vi "MFLI controller -- via frontend -- V2.vi"(1 "MFLI controller action":T1=enum."Scan frequency", 5 "Address":string="DEV3523", 9 "sweep parameters":T2={"scan type"=enum."arctan", "N"=100, "cursor window"={"left"=32571.699125630872, "right "=32589.533031344432, "center"=32580.616078487652, "window"=17.83390571355876, "cursors"=[0, 1, 2], "relative"=0, "absolute"=0, "fixed vertical offset"=0.0, "vertical offset"=0.0, "skew"=0.0, "default window frac"=0.1, "kind"=enum."symmetric", "skew.left"=0.5, "skew.right"=0.5, "Plot ref"=refnum, "wing order"=enum."forw"}}, 11 "Error In":errorcluster, 12 "reqested size":i32=100, 13 "delay (msec)":i64=2) -> (4 "Freq out (Hz)":dbl[](array[numeric])=[32012.991918577427, 32390.261658505893, 32466.39798177853, 32499.14340521798, 32517.39286113775, 32529.046092051318, 32537.14525712326, 32543.111142615544, 32547.696343954158, 32551.33675949651, 32554.302325209504, 32556.769142360055, 32558.856995237307, 32560.650202739795, 32562.209843476354, 32563.58125099723, 32564.7987833122, 32565.88895894197, 32566.872575330308, 32567.766175404246, 32568.583086316496, 32569.334166794306, 32570.02835688638, 32570.673085530187, 32571.274580490695, 32571.838104118455, 32572.36813539066, 32572.868514009202, 32573.342552524307, 32573.793126289274, 32574.222746575288, 32574.633618125405, 32575.027687968828, 32575.40668442971, 32575.772149741057, 32576.12546690325, 32576.467883345118, 32576.800529469096, 32577.124435064776, 32577.440543590797, 32577.749724325146, 32578.052781957467, 32578.35046682089, 32578.643482565894, 32578.932492128843, 32579.218126471686, 32579.500987779396, 32579.781656707495, 32580.06069600583, 32580.338656060805, 32580.616078519142, 32580.89350097748, 32581.171461032456, 32581.45050033079, 32581.73116925889, 32582.0140305666, 32582.29966469628, 32582.58867447239, 32582.88169000423, 32583.179375080817, 32583.48243271314, 32583.791613234323, 32584.10772197351, 32584.43162756919, 32584.764273480003, 32585.106690135035, 32585.460007297228, 32585.825472395412, 32586.204468856296, 32586.59853891288, 32587.009410462997, 32587.439030535847, 32587.889604513977, 32588.363642815923, 32588.86402143446, 32589.39405291983, 32589.957576334426, 32590.559071508098, 32591.203800151903, 32591.897990030815, 32592.64907072179, 32593.46598163404, 32594.359581707977, 32595.343197883154, 32596.433373726086, 32597.650906041054, 32599.022313348767, 32600.58195429849, 32602.375161800977, 32604.46301467823, 32606.929831615616, 32609.895397541775, 32613.535812870963, 32618.12101442274, 32624.086899701866, 32632.186064986967, 32643.839295900536, 32662.088751820305, 32694.834175046595, 32770.97049853239], 6 "sweep time":dbl=1.133070214302279, 10 "Voltage out (V)":cdb[](array[numeric])=[1.7183506006211996e-05-0.0001154032788780638i, 1.7124360968751133e-05-0.0001154114779288915i, 1.7049104347380084e-05-0.00011541542942613611i, 1.700437896335042e-05-0.00011541749156201827i, 1.6984579723285106e-05-0.00011542204741013496i, 1.702277369054923e-05-0.00011543195548892015i, 1.713094025845651e-05-0.00011543928112855599i, 1.734249707866828e-05-0.00011543960094139092i, 1.768320429215342e-05-0.0001154245402225022i, 1.8195281152538477e-05-0.00011538335923575508i, 1.8917228661806973e-05-0.00011530288392402138i, 1.9897834564883332e-05-0.00011516640933089982i, 2.154104046962704e-05-0.0001148906117047364i, 2.3247799321765792e-05-0.00011455940834964969i, 2.5364678450551808e-05-0.00011410149936074356i, 2.8645788781885885e-05-0.00011331572480450341i, 3.204749554800641e-05-0.00011242961468546203i, 3.783559691555022e-05-0.00011080033368711338i, 4.245015867332296e-05-0.00010941815048749576i, 4.909131821431355e-05-0.0001073312840925185i, 5.511821898441184e-05-0.00010535829212367013i, 6.178843506022867e-05-0.00010310289174359778i, 7.1079604965352e-05-9.985157907779013e-05i, 7.922304381453334e-05-9.690255343156676e-05i, 8.814778883893872e-05-9.35627973091444e-05i, 9.806709148886077e-05-8.971246458508318e-05i, 0.00011119043245647465-8.437841897470898e-05i, 0.00012253184919712196-7.953180105990741e-05i, 0.00013777724317049346-7.26422052575784e-05i, 0.0001508081004573332-6.638511645494567e-05i, 0.00016547294918783876-5.890291826790314e-05i, 0.00018003847596605868-5.097295421607585e-05i, 0.00019518361086534857-4.2160672625888326e-05i, 0.00021134179818259658-3.207632261667366e-05i, 0.0002372041782935464-1.434566976209705e-05i, 0.00025518143132024254-7.65423157605567e-07i, 0.0002835129702467886+2.297908707067173e-05i, 0.0003060118087631287+4.414715126576145e-05i, 0.00032860772064336976+6.780161699354136e-05i, 0.0003492674091322389+9.188627597766353e-05i, 0.00037498324855458583+0.0001258445655672888i, 0.00040021078021115026+0.00016463936720210011i, 0.00041969942568205823+0.0001996255883353531i, 0.00044367338947118773+0.00025154867300893595i, 0.0004634793607238068+0.0003068834938295352i, 0.00047921028781215815+0.00036805191402776324i, 0.0004880906353641744+0.00042166295770603194i, 0.0004932212623741357+0.0004947057496862386i, 0.000491476456593048+0.0005562791342814882i, 0.000480893803992059+0.0006363872629062725i, 0.0004535995818650303+0.0007373086546111893i, 0.000417087772881063+0.0008226852134031236i, 0.0003564148692854789+0.0009214817173403453i, 0.0003049201646356487+0.0009841224100520793i, 0.00021260191240459413+0.0010684135492785532i, 0.00011714858948470126+0.001130293664798013i, 1.675457544365132e-05+0.0011752384955043165i, -6.8674075405897e-05+0.0012001399159748158i, -0.000156473047607305+0.0012143601357779102i, -0.00026709373934749337+0.0012167952520739987i, -0.0003544271565676041+0.001206585218500233i, -0.00047937600197311275+0.0011721904461218277i, -0.0006086290582260493+0.0011080263068835828i, -0.0007031877411848573+0.0010369948237613604i, -0.0007564526901441745+0.0009845652865779295i, -0.000802489180995596+0.0009292050493656664i, -0.0008414596018105983+0.0008721985101652608i, -0.0008809346482248761+0.0008000538120167723i, -0.0009073902840241921+0.0007382113118499092i, -0.0009264953054508651+0.000680980624166274i, -0.0009405659412141811+0.0006247883223244968i, -0.000951649722530156+0.0005564170049287236i, -0.0009557485581057351+0.0005027508202624884i, -0.0009558464741053665+0.0004515634249715623i, -0.0009509110176922098+0.0003899637122391104i, -0.0009411315169847015+0.00033238768338539245i, -0.0009303400913929496+0.0002890952314710416i, -0.0009171113529290538+0.00024772942260094455i, -0.0009022111527275027+0.00020961974320628598i, -0.0008813746494947608+0.00016554205395646727i, -0.0008581837971946129+0.00012481593212717478i, -0.0008372063466683705+9.328565348151487e-05i, -0.0008165626610594428+6.595676342721183e-05i, -0.0007901155435838691+3.51376371228606e-05i, -0.0007682834352800848+1.2585785624721776e-05i, -0.000746231015527196-7.956667433689733e-06i, -0.0007238798463130141-2.6771164006128246e-05i, -0.0007015567569177018-4.3779400880525094e-05i, -0.000679301954671598-5.9154880569231366e-05i, -0.0006572001413831251-7.301304884663801e-05i, -0.000629855254567978-8.838260380910578e-05i, -0.0006083942229188815-9.917719243438264e-05i, -0.0005768631156754208-0.00011317657292622015i, -0.0005562177438951648-0.00012121832857134644i, -0.0005359092039599222-0.00012831021292074535i, -0.0005145186443378148-0.00013494179211461784i, -0.0004951602053444319-0.00014023403510992087i, -0.00047624970229075174-0.00014478034103386663i, -0.0004577401041527736-0.00014865456703421655i, -0.00043519037796120065-0.00015262867452433312i])   [LabVIEW 2017]
uses:
  sweep parameters.ctl
  cursor winow.ctl
  MFLI controller action.ctl
  publisher action.ctl
panel:
  out "scan progress":i32(slide) min=0 max=257 scale=0.0..257.0
  out "ind":i64=42
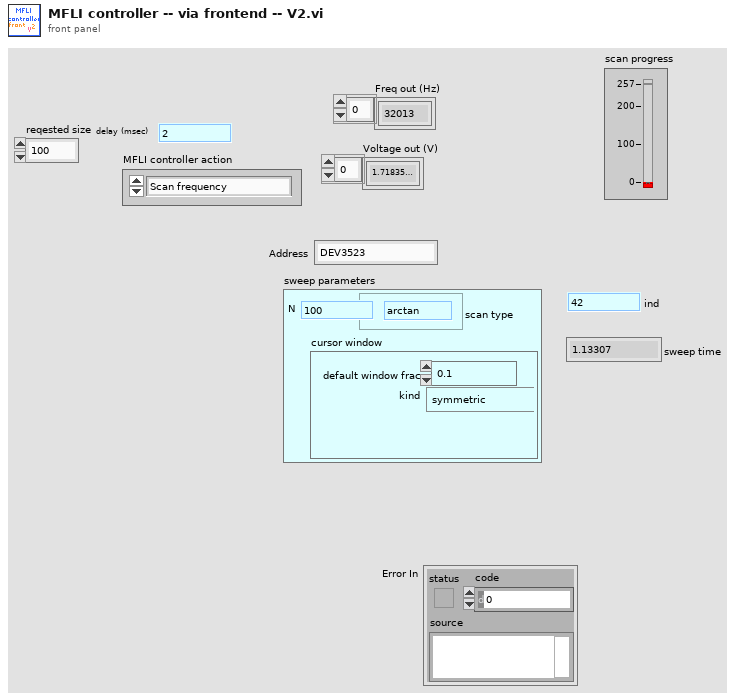
[diagram p1: front panel]
types:
  T1 = typedef "MFLI controller action.ctl" = enum16{"Initialize", "Scan frequency", "open", "close", "read", "circle PLL"}
  T2 = typedef "sweep parameters.ctl" = cluster{"scan type":enum16{"linear", "arctan"}, "N":i64, "cursor window":T3}
  T3 = typedef "cursor winow.ctl" = cluster{"left":dbl, "right ":dbl, "center":dbl, "window":dbl, "cursors":i32[], "relative":i32, "absolute":i32, "fixed vertical offset":dbl, "vertical offset":dbl, "skew":dbl, "default window frac":dbl, "kind":enum16{"symmetric", "skewed", "fancy"}, "skew.left":dbl, "skew.right":dbl, "Plot ref":refnum<vi>, "wing order":enum16{"forw", "back"}}
  T4 = typedef "publisher action.ctl" = enum16{"set", "get"}
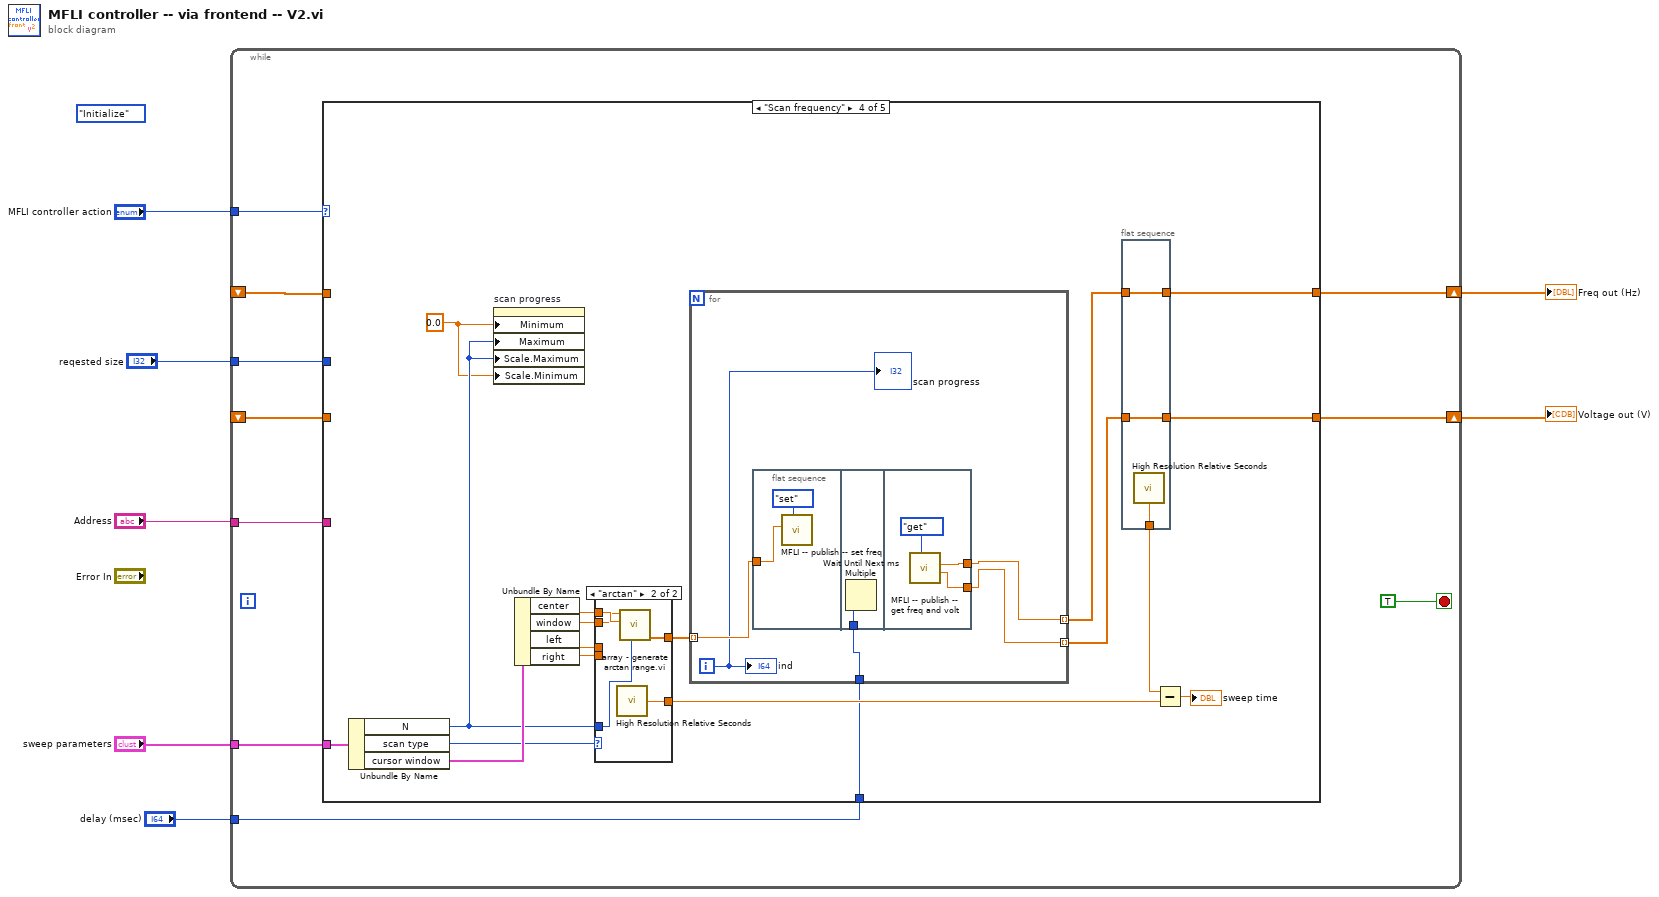
[diagram p0: block diagram]
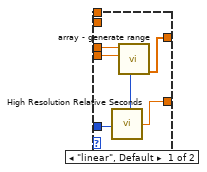
[diagram p5: hidden frame]
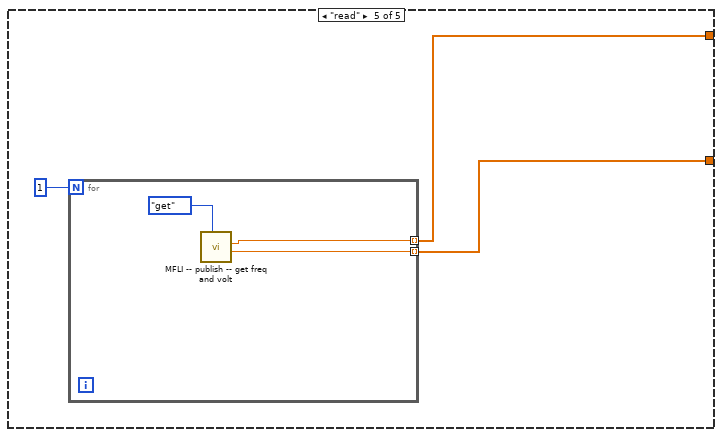
[diagram p6: hidden frame]
diagram:
  (unwired) MFLI_controller_action."Initialize" ("MFLI controller action")
  n1 = while {
    shift-right: [w17] -> w7
    shift-left: _ -> [w15]
    shift-right: [w16] -> w6
    shift-left: _ -> [w14]
    tunnel: "MFLI controller action" -> [w12]
    tunnel: "sweep parameters" -> [w11]
    tunnel: "Address" -> [w10]
    tunnel: "reqested size" -> [w9]
    tunnel: "delay (msec)" -> [w8]
    stop <- TRUE stop-if-true
    n2 = case shown="\"Scan frequency\"" w12 {
      tunnel: [w19 w21 w23 w41 w66] -> w17
      tunnel: [w18 w20 w22 w40 w67] -> w16
      tunnel: w15 -> [w19 w21 w23 _ _]
      tunnel: w14 -> [w18 w20 w22 _ _]
      tunnel: w11 -> [_ _ _ w29 _]
      tunnel: w10 -> [_ _ _ _ _]
      tunnel: w9 -> [_ _ _ _ _]
      tunnel: w8 -> [_ _ _ w26 _]
      frame "Initialize", Default {
      }
      frame "open" {
      }
      frame "close" {
        # "close Device"
      }
      frame "Scan frequency" {
        w24 = 0.0 ("Data Entry Limits:Minimum")
        n3 = Unbundle By Name(w29) -> ("N"=w25:i64, "scan type"=w27:enum16{"linear", "arctan"}, "cursor window"=w28:T3)
        n4 = property on="scan progress" class="Slide (strict)"("Minimum"=w24, "Maximum"=w25, "Scale.Maximum"=w25, "Scale.Minimum"=w24) -> ()  [unwired: 2 in, 2 out]
        n5 = Unbundle By Name(w28) -> ("center"=w36:dbl, "window"=w35:dbl, "left"=w34:dbl, "right"=w33:dbl)
        n6 = case shown="\"arctan\"" w27 {
          tunnel: [w46 w51] -> w39
          tunnel: w36 -> [_ w50]
          tunnel: w35 -> [_ w49]
          tunnel: w34 -> [w45 _]
          tunnel: w33 -> [w44 _]
          tunnel: [w43 w48] -> w32
          tunnel: w25 -> [w42 w47]
          frame "linear", Default {
            n7 = call <vilib>:"High Resolution Relative Seconds.vi"() -> ("relative seconds"=w43:dbl)
            n8 = call "array - generate range.vi"("N"=w42, "freq max"=w44, "freq min"=w45) -> ("Array"=w46:dbl[])  [unwired: 7 in, 1 out]
          }
          frame "arctan" {
            n9 = call <vilib>:"High Resolution Relative Seconds.vi"() -> ("relative seconds"=w48:dbl)
            n10 = call "array - generate arctan range.vi.vi"("N"=w47, "omega0"=w50, "gamma"=w49) -> ("Array"=w51:dbl[])  [unwired: 8 in]
          }
        }
        n11 = for {
          tunnel: w39 -> [w56] mode=indexing
          tunnel: [w54] -> w38 mode=indexing
          tunnel: [w53] -> w37 mode=indexing
          tunnel: w26 -> [w55]
          i -> [w52]
          n12 = flat-sequence {
            tunnel: w56 -> [w58]
            tunnel: w55 -> [w59]
            tunnel: [w62] -> w54
            tunnel: [w61] -> w53
            frame #0 {
              n13 = call "MFLI -- publish -- set freq.vi"("publisher action"=publisher_action."set", "freq IN (Hz)"=w58) -> ()  [unwired: 9 in, 1 out]
            }
            frame #1 {
              n14 = Wait Until Next ms Multiple(millisecond multiple=w59) -> ()  [unwired: 1 out]
            }
            frame #2 {
              n15 = call "MFLI -- publish -- get freq and volt.vi"("publisher action"=publisher_action."get") -> ("Voltage out (V)"=w61:cdb, "freq out (Hz)"=w62:dbl)  [unwired: 9 in]
            }
          }
          "ind" <- w52
          "scan progress" <- w52
        }
        n16 = flat-sequence {
          tunnel: w38 -> [w65]
          tunnel: [w65] -> w41
          tunnel: w37 -> [w64]
          tunnel: [w64] -> w40
          tunnel: [w63] -> w31
          frame #0 {
            n17 = call <vilib>:"High Resolution Relative Seconds.vi"() -> ("relative seconds"=w63:dbl)
          }
        }
        n18 = Subtract(x=w31, y=w32) -> (x-y=→"sweep time":dbl)
      }
      frame "read" {
        n19 = for {
          N: 1 -> [_]
          tunnel: [w70] -> w66 mode=indexing
          tunnel: [w69] -> w67 mode=indexing
          n20 = call "MFLI -- publish -- get freq and volt.vi"("publisher action"=publisher_action."get") -> ("Voltage out (V)"=w69:cdb, "freq out (Hz)"=w70:dbl)  [unwired: 9 in]
        }
      }
    }
  }
  "Freq out (Hz)" <- w7
  "Voltage out (V)" <- w6
